vi "Dual Interval Signal.vi"(0 "Enable?":bool, 1 "Delay":dbl, 2 "On Time":dbl, 3 "Off Time":dbl) -> (4 "Output":bool)   [LabVIEW 2016]
uses:
  Change Detect Boolean.vi
panel:
  # "because james' is confusing"
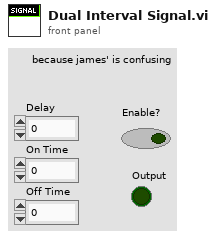
[diagram p1: front panel]
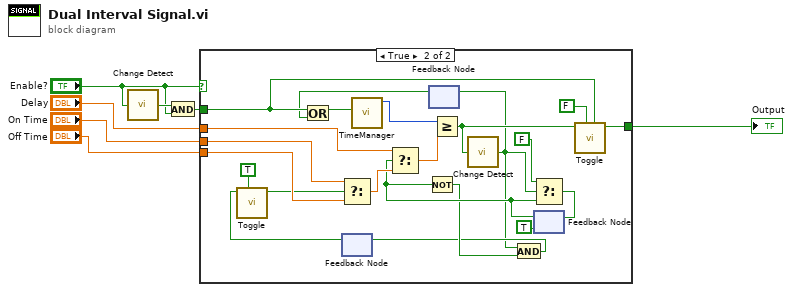
[diagram p0: block diagram]
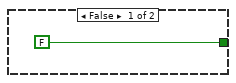
[diagram p2: hidden frame]
diagram:
  n1 = call-poly "Change Detect.vi"("In"="Enable?") -> ("Changed?"=w7:bool)
  n2 = And(x=w7, y="Enable?") -> (x .and. y?=w2:bool)
  n3 = case shown="True" "Enable?" {
    tunnel: w2 -> [_ w20]
    tunnel: "Delay" -> [_ w28]
    tunnel: "On Time" -> [_ w26]
    tunnel: "Off Time" -> [_ w25]
    tunnel: [FALSE ("Toggled") w22] -> w3
    frame False {
    }
    frame True {
      n4 = feedback #1() -> (w12:bool)  [unwired: 1 in]
      n5 = call "Toggle.vi"("Initial Value"=TRUE, "In"=w12) -> ("Toggled"=w24:bool)  [unwired: 9 in]
      n6 = Select(t=w26, s=w24, f=w25) -> (s? t:f=w27:dbl)
      n7 = feedback #2() -> (w9:bool)  [unwired: 1 in]
      n8 = Or(x=w20, y=w9) -> (x .or. y?=w11:bool)
      n9 = call "TimeManager.vi"("Reset?"=w11) -> ("Time Since Reset"=w29:u32)  [unwired: 9 in, 1 out]
      n10 = feedback #3(TRUE) -> (w15:bool)
      n11 = Select(t=w28, s=w15, f=w27) -> (s? t:f=w30:dbl)
      n12 = Not(x=w15) -> (.not. x?=w14:bool)
      n13 = Greater Or Equal?(x=w29, y=w30) -> (x >= y?=w16:bool)
      n14 = call-poly "Change Detect.vi"("In"=w16) -> ("Changed?"=w10:bool)
      n15 = feedback-in #2(w10) -> ()
      n16 = And(x=w10, y=w14) -> (x .and. y?=w13:bool)
      n17 = feedback-in #1(w13) -> ()
      n18 = Select(t=FALSE, s=w10, f=w15) -> (s? t:f=w18:bool)
      n19 = feedback-in #3(w18) -> ()
      n20 = call "Toggle.vi"("Reinit?"=w20, "Initial Value"=FALSE, "In"=w16) -> ("Toggled"=w22:bool)  [unwired: 8 in]
    }
  }
  "Output" <- w3
